vi "ep_Check dt (N Channels).vi"(7 "reset? (F)":bool, 8 "error in (no error)":errorcluster, 10 "waveforms only? (F)":bool, 11 "waveforms":waveform(dbl)[](array[waveform])) -> (0 "error out":errorcluster, 1 "dup waveforms":waveform(dbl)[](array[waveform]), 2 "dt":dbl, 3 "signals":dbl[][](array[numeric]), 5 "t0":timestamp)   [LabVIEW 2013, in "NI_EP_Power Measurement.lvlib"]
uses:
  <vilib>/addons/Electrical Power/Power Measurement/NI_EP_Power Measurement.lvlib
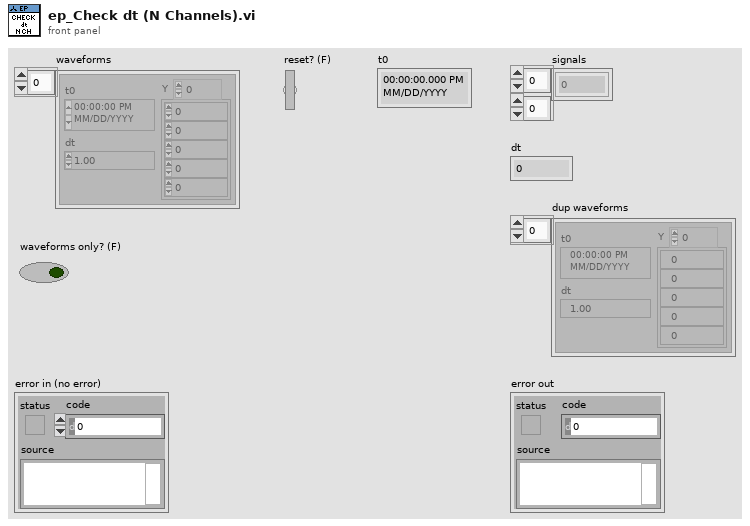
[diagram p1: front panel]
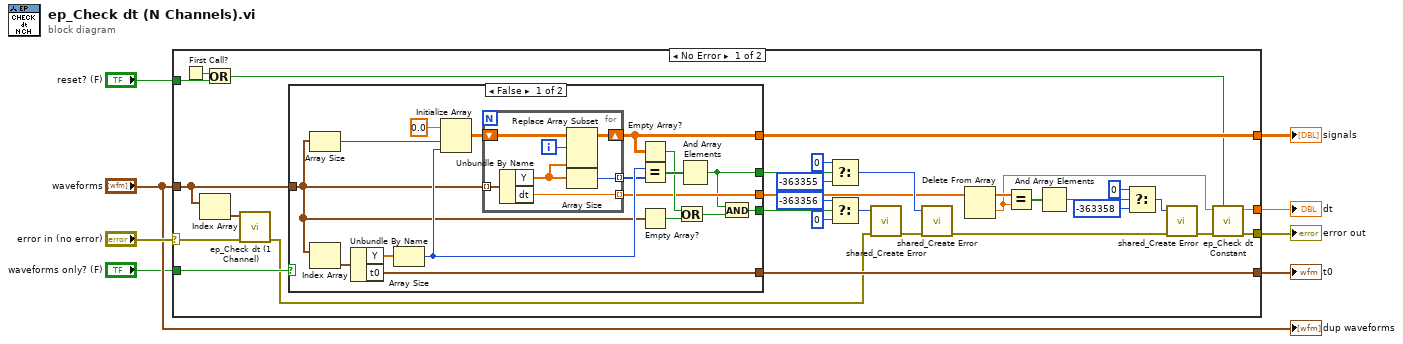
[diagram p0: block diagram]
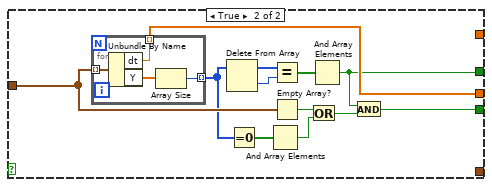
[diagram p2: hidden frame]
diagram:
  n1 = case shown="No Error" "error in (no error)" {
    selector: "error in (no error)" -> [w14 w80]
    tunnel: "waveforms" -> [w12 _]
    tunnel: [w19 w80] -> w7
    tunnel: [w38 _] -> w6
    tunnel: [w39 _] -> w5
    tunnel: [w18 _] -> w3
    tunnel: "reset? (F)" -> [w15 _]
    tunnel: "waveforms only? (F)" -> [w37 _]
    frame No Error {
      n2 = First Call?() -> (First Call?: T/F=w17:bool)
      n3 = Index Array(array=w12) -> (element=w13:waveform(dbl))  [unwired: 1 in]
      n4 = Or(x=w17, y=w15) -> (x .or. y?=w16:bool)
      n5 = call <vilib>:"ep_Check dt (1 Channel).vi"("error in (no error)"=w14, "waveform in"=w13) -> ("error out"=w11:errorcluster)  [unwired: 8 in, 1 out]
      n6 = case shown="False" w37 {
        tunnel: [w56 _] -> w39
        tunnel: [w50 _] -> w38
        tunnel: w12 -> [w46 w73]
        tunnel: [w42 w66] -> w23
        tunnel: [w41 w65] -> w22
        tunnel: [w40 w64] -> w21
        frame False {
          n7 = Array Size(array=w46) -> (size(s)=w55:i32)
          n8 = Index Array(array=w46) -> (element=w52:waveform(dbl))  [unwired: 1 in]
          n9 = Unbundle By Name(w52) -> ("Y"=w51:dbl[], "t0"=w56:timestamp)
          n10 = Array Size(array=w51) -> (size(s)=w48:i32)
          n11 = Initialize Array(0.0 ("element"), w55, w48) -> (w53:dbl[][])
          n12 = for {
            tunnel: w46 -> [w63] mode=indexing
            tunnel: [w62] -> w42 mode=indexing
            shift-right: [w59] -> w50
            shift-left: w53 -> [w61]
            tunnel: [w57] -> w44 mode=indexing
            i -> [w60]
            n13 = Unbundle By Name(w63) -> ("Y"=w58:dbl[], "dt"=w62:dbl)
            n14 = Replace Array Subset(array=w61, new element=w58, index (row)=w60) -> (w59:dbl[][])  [unwired: 1 in]
            n15 = Array Size(array=w58) -> (size(s)=w57:i32)
          }
          n16 = Empty Array?(array=w50) -> (empty?=w47:bool)
          n17 = Equal?(x=w48, y=w44) -> (x = y?=w49:bool[])
          n18 = Empty Array?(array=w46) -> (empty?=w45:bool)
          n19 = Or(x=w47, y=w45) -> (x .or. y?=w43:bool)
          n20 = And Array Elements(Boolean array=w49) -> (logical AND=w40:bool)
          n21 = And(x=w40, y=w43) -> (x .and. y?=w41:bool)
        }
        frame True {
          n22 = for {
            tunnel: w73 -> [w79] mode=indexing
            tunnel: [w78] -> w69 mode=indexing
            tunnel: [w76] -> w66 mode=indexing
            n23 = Unbundle By Name(w79) -> ("dt"=w76:dbl, "Y"=w77:dbl[])
            n24 = Array Size(array=w77) -> (size(s)=w78:i32)
          }
          n25 = Delete From Array(array=w69) -> (deleted portion=w71:i32, array with subset deleted=w72:i32[])  [unwired: 2 in]
          n26 = Equal To 0?(x=w69) -> (x = 0?=w70:bool[])
          n27 = And Array Elements(Boolean array=w70) -> (logical AND=w67:bool)
          n28 = Equal?(x=w72, y=w71) -> (x = y?=w75:bool[])
          n29 = Empty Array?(array=w73) -> (empty?=w68:bool)
          n30 = Or(x=w68, y=w67) -> (x .or. y?=w74:bool)
          n31 = And Array Elements(Boolean array=w75) -> (logical AND=w64:bool)
          n32 = And(x=w64, y=w74) -> (x .and. y?=w65:bool)
        }
      }
      n33 = Select(t=0, s=w21, f=-363355) -> (s? t:f=w24:i32)
      n34 = Select(t=-363356, s=w22, f=0) -> (s? t:f=w30:i32)
      n35 = call <vilib>:"shared_Create Error.vi"("error in (no error)"=w11, "error code (0)"=w30) -> ("error out"=w25:errorcluster)  [unwired: 9 in]
      n36 = call <vilib>:"shared_Create Error.vi"("error in (no error)"=w25, "error code (0)"=w24) -> ("error out"=w20:errorcluster)  [unwired: 9 in]
      n37 = Delete From Array(array=w23) -> (deleted portion=w9:dbl, array with subset deleted=w10:dbl[])  [unwired: 2 in]
      n38 = Equal?(x=w10, y=w9) -> (x = y?=w36:bool[])
      n39 = And Array Elements(Boolean array=w36) -> (logical AND=w35:bool)
      n40 = Select(t=0, s=w35, f=-363358) -> (s? t:f=w32:i32)
      n41 = call <vilib>:"shared_Create Error.vi"("error in (no error)"=w20, "error code (0)"=w32) -> ("error out"=w31:errorcluster)  [unwired: 9 in]
      n42 = call <vilib>:"ep_Check dt Constant.vi"("reset? (F)"=w16, "error in (no error)"=w31, "dt"=w9) -> ("error out"=w19:errorcluster, "dup dt"=w18:dbl)  [unwired: 7 in]
    }
    frame Error {
    }
  }
  "error out" <- w7
  "signals" <- w6
  "dt" <- w3
  "t0" <- w5
  "dup waveforms" <- "waveforms"
